vi "Read_tcx_file.vi"(7 "Path":path, 8 "error in (no error)":errorcluster, 11 "HR Data Structure":T1) -> (0 "error out":errorcluster, 3 "HR Data Structure 2":T1)   [LabVIEW 2021]
uses:
  HR Data Structure.ctl
  Runner's Data.ctl
  Raw Data.ctl
  <vilib>/Utility/file.llb/Read Delimited Spreadsheet (string).vi
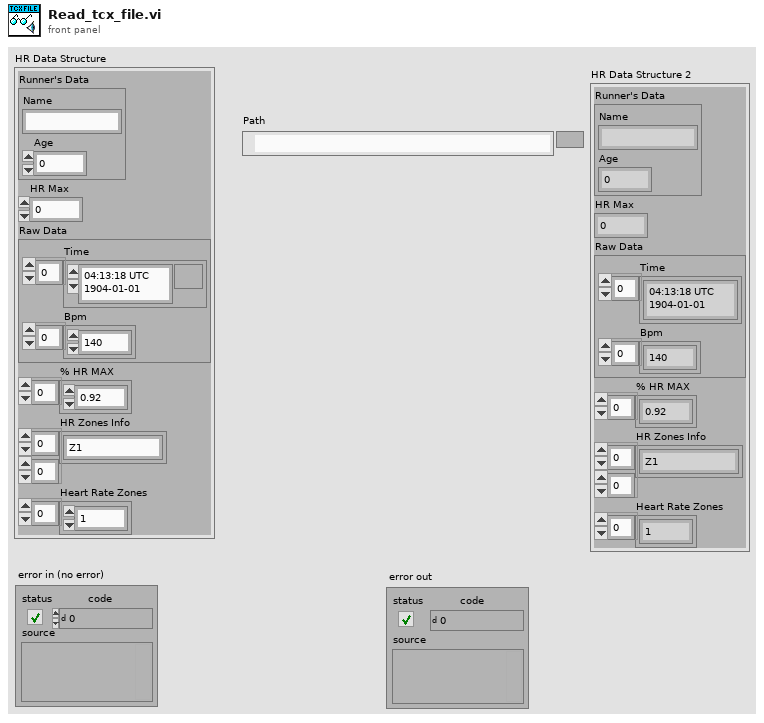
[diagram p1: front panel]
types:
  T1 = typedef "HR Data Structure.ctl" = cluster{"Runner's Data":T2, "HR Max":i32, "Raw Data":T3, "% HR MAX ":dbl[], "HR Zones Info":string[][], "Heart Rate Zones":dbl[]}
  T2 = typedef "Runner's Data.ctl" = cluster{"Name":string, "Age":i32}
  T3 = typedef "Raw Data.ctl" = cluster{"Time":timestamp[], "Bpm":i32[]}
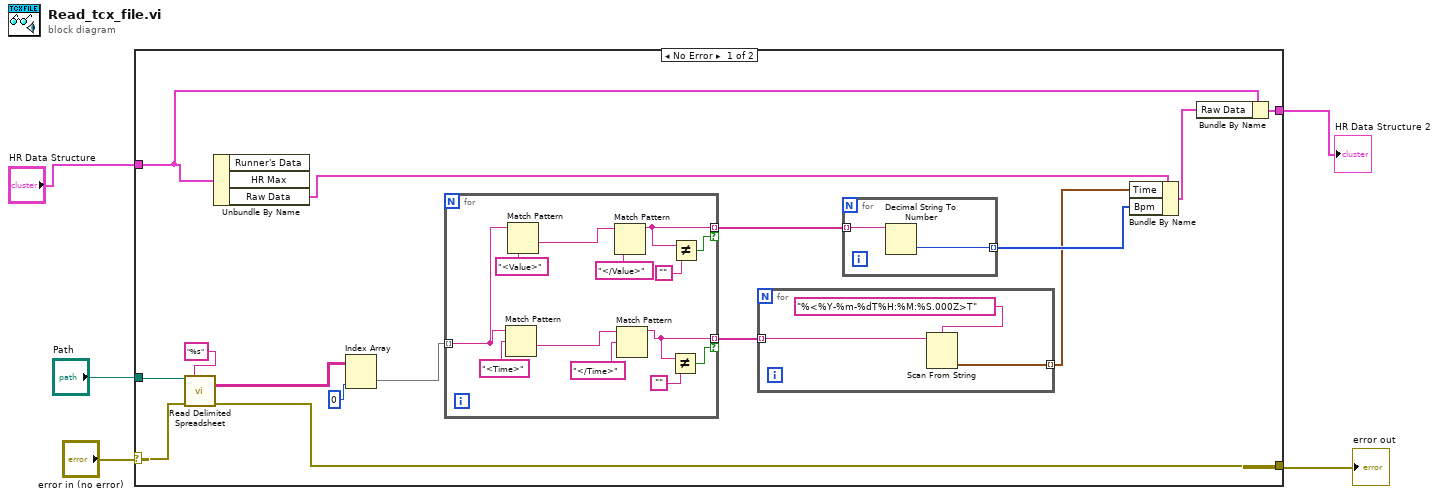
[diagram p0: block diagram]
diagram:
  n1 = case shown="No Error" "error in (no error)" {
    selector: "error in (no error)" -> [w20 w39]
    tunnel: [w19 w39] -> w4
    tunnel: "HR Data Structure" -> [w11 w40]
    tunnel: [w9 w40] -> w2
    tunnel: "Path" -> [w8 _]
    frame No Error {
      n2 = call-poly <vilib>:"Read Delimited Spreadsheet.vi"("file path (dialog if empty)"=w8, "format (%s)"="%s", "error in (no error)"=w20) -> ("all rows"=w17:string[][], "error out"=w19:errorcluster)  [unwired: 7 in, 4 out]
      n3 = Unbundle By Name(w11) -> ("Raw Data"=w14:T3)  [unwired: 2 out]
      n4 = Index Array(array=w17, index (col)=0 ("disabled index (col)")) -> (element=w7:string[])  [unwired: 1 in]
      n5 = for {
        tunnel: w7 -> [w38] mode=indexing
        tunnel: [w29] -> w16 mode=indexing if=w28
        tunnel: [w27] -> w15 mode=indexing if=w26
        n6 = Match Pattern(string=w38, regular expression="<Time>") -> (after substring=w36:string)  [unwired: 1 in, 3 out]
        n7 = Match Pattern(string=w38, regular expression="<Value>") -> (after substring=w33:string)  [unwired: 1 in, 3 out]
        n8 = Match Pattern(string=w33, regular expression="</Value>") -> (before substring=w29:string)  [unwired: 1 in, 3 out]
        n9 = Match Pattern(string=w36, regular expression="</Time>") -> (before substring=w27:string)  [unwired: 1 in, 3 out]
        n10 = Not Equal?(x=w27, y="") -> (x != y?=w26:bool)
        n11 = Not Equal?(x=w29, y="") -> (x != y?=w28:bool)
      }
      n12 = for {
        tunnel: w15 -> [w22] mode=indexing
        tunnel: [w21] -> w12 mode=indexing
        n13 = Scan From String(format string="%<%Y-%m-%dT%H:%M:%S.000Z>T", input string=w22) -> (output 1=w21:timestamp)  [unwired: 3 in, 3 out]
      }
      n14 = for {
        tunnel: w16 -> [w25] mode=indexing
        tunnel: [w24] -> w13 mode=indexing
        n15 = Decimal String To Number(string=w25) -> (number=w24:i32)  [unwired: 2 in, 1 out]
      }
      n16 = Bundle By Name(cluster=w14, "Time"=w12, "Bpm"=w13) -> (w10:T3)
      n17 = Bundle By Name(cluster=w11, "Raw Data"=w10) -> (w9:T1)
    }
    frame Error {
    }
  }
  "error out" <- w4
  "HR Data Structure 2" <- w2
